vi "Test Set Subpanels-- SMO Array.vi"(8 "error in":errorcluster) -> (0 "error out":errorcluster)   [LabVIEW 2020]
uses:
  <vilib>/addons/_JKI Toolkits/Caraya/classes/Test/Test.lvclass
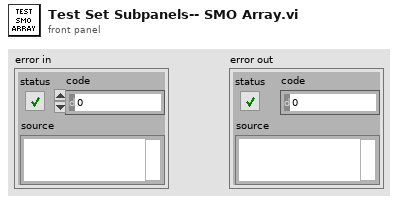
[diagram p1: front panel]
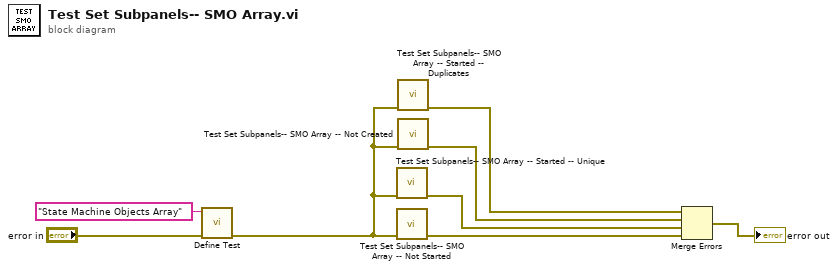
[diagram p0: block diagram]
diagram:
  n1 = call <vilib>:"Define Test.vi"("error in (no error)"="error in", "Label (VI Title)"="State Machine Objects Array") -> ("error out"=w2:errorcluster)  [unwired: 9 in]
  n2 = call "Test Set Subpanels-- SMO Array -- Started -- Unique.vi"("error in"=w2) -> ("error out"=w4:errorcluster)  [unwired: 10 in]
  n3 = call "Test Set Subpanels-- SMO Array -- Not Started.vi"("error in"=w2) -> ("error out"=w5:errorcluster)  [unwired: 10 in]
  n4 = call "Test Set Subpanels-- SMO Array -- Started -- Duplicates.vi"("error in"=w2) -> ("error out"=w1:errorcluster)  [unwired: 10 in]
  n5 = call "Test Set Subpanels-- SMO Array -- Not Created.vi"("error in"=w2) -> ("error out"=w3:errorcluster)  [unwired: 10 in]
  n6 = Merge Errors(w1, w3, w4, w5) -> (→"error out":errorcluster)
